vi "TETS Query IPG.vi"(0 "Command":T1(ring), 11 "error in":errorcluster) -> (4 "Response Byte":u8, 15 "error out":errorcluster)   [LabVIEW 2010]
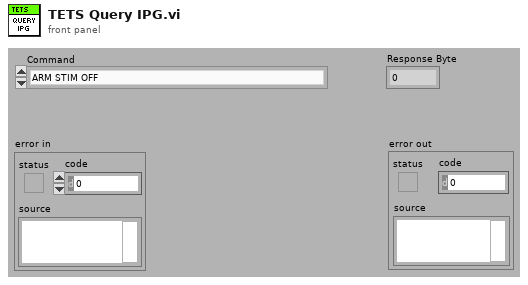
[diagram p1: front panel]
types:
  T1 = enum8{"ARM STIM OFF", "STIM OFF", "(unused1)", "GET IPG STATUS - GEN BYTE", "GET IPG STATUS - SELECTED PROGRAM", "CHARGE OFF", "(unused2)", "CHARGE CONTROL - VRECT", "CHARGE CONTROL - STATE/TEMP", "GET IPG STATUS - BATTERY STATE", "GET IPG STATUS - ACTIVE ERROR BYTE", "GET IPG STATUS - CHARGING ERROR BYTE", "ARM PAIR POP", "ARM PAIR PPC", "(unused3)", "(unused4)"}
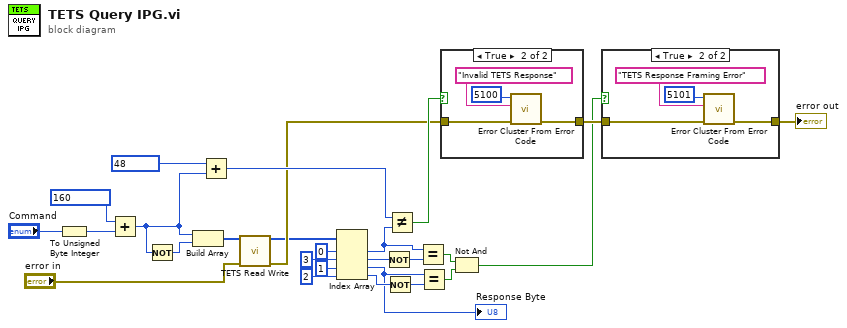
[diagram p0: block diagram]
diagram:
  n1 = To Unsigned Byte Integer(number="Command") -> (unsigned 8bit integer=w26:u8)
  n2 = Add(x=u8 160, y=w26) -> (x+y=w13:u8)
  n3 = Not(x=w13) -> (.not. x?=w24:u8)
  n4 = Build Array(w13, w24) -> (w2:u8[])
  n5 = Add(x=u8 48, y=w13) -> (x+y=w10:u8)
  n6 = call "TETS Read Write.vi"("Input Bytes"=w2, "error in"="error in") -> ("Output Bytes"=w1:u8[], "error in"=w4:errorcluster)  [unwired: 12 in]
  n7 = Index Array(array=w1, index #1=0 ("index"), index #2=3 ("index"), index #3=1 ("index"), index #4=2 ("index")) -> (element #1=w11:u8, element #2=w19:u8, element #3=w9:u8, element #4=w16:u8)
  "Response Byte" <- w9
  n8 = Not(x=w19) -> (.not. x?=w18:u8)
  n9 = Not(x=w16) -> (.not. x?=w17:u8)
  n10 = Not Equal?(x=w10, y=w11) -> (x != y?=w6:bool)
  n11 = Equal?(x=w11, y=w18) -> (x = y?=w15:bool)
  n12 = Equal?(x=w9, y=w17) -> (x = y?=w14:bool)
  n13 = case shown="True" w6 {
    tunnel: [w28 w30] -> w8
    tunnel: w4 -> [w28 w29]
    frame False {
    }
    frame True {
      n14 = call <vilib>:"Error Cluster From Error Code.vi"("error in (no error)"=w29, "error message (\"\")"="Invalid TETS Response" ("error message (\"\")"), "error code (0)"=5100) -> ("error out"=w30:errorcluster)  [unwired: 6 in]
    }
  }
  n15 = Not And(1:w14, 2:w15) -> (0:w5:bool)
  n16 = case shown="True" w5 {
    tunnel: w8 -> [w33 w35]
    tunnel: [w33 w34] -> w7
    frame False {
    }
    frame True {
      n17 = call <vilib>:"Error Cluster From Error Code.vi"("error in (no error)"=w35, "error message (\"\")"="TETS Response Framing Error" ("error message (\"\")"), "error code (0)"=5101) -> ("error out"=w34:errorcluster)  [unwired: 6 in]
    }
  }
  "error out" <- w7
